vi "Module for RF and LO synthesizer.vi"(10 "Main controller mailbox":T4, 11 "THz module mailbox":T4) -> ()   [LabVIEW 2021, in "THz source modeule.lvlib"]
doc: "Module to set constant frequency or simple frequency sweep on RF (main) synthesizer and offset frequency on LO (folowing) synthesizer.\nKey typedefs: THz_Message for module, THz_Comands enum (Ignore, Initialize, Update, Set parameters, Disconnect, End), THz_Sweeep parameters\n\nComands and responses:\nInitialize: VDI config constants {Master{lower limit, upper limit, name, handle, description}, Follower{ lower limit, upper limit, name, handle, description } } (cluster of two clusters {numeric, numeric, string, numeric, string}) / handle log (string)\nUpdate: - / M_ID F_ID (string)\nSet parameters: Sweep parameters {Start, End, Sweep up time, Sweep down time, Intermediate, Reset trigger} (cluster{numeric, numeric, numeric, numeric, numeric, boolean}) / Sweep parameters (same cluster)\nDisconnect: - / master and follower name (string)\nEnd: - / Master and Follower handle (string)"
uses:
  THz source modeule.lvlib
  Messenger service/Data types/Mailbox address.ctl
  ctl/VDI config constants.ctl
  ctl/Synth configs.ctl
  ctl/THz sweep parameters.ctl
  Messenger service/Data types/Module name.ctl
  ctl/THz Message for module.ctl
  ctl/THz commands enum.ctl
  <vilib>/Utility/error.llb/Error Cluster From Error Code.vi
  <vilib>/ErrorRing/Error Ring.xnode
  Messenger service/MessengerLib.lvlib
panel:
  out "FT_Status_Update_Master":u32(ring) items=["FT_OK", "FT_INVALID_HANDLE", "FT_DEVICE_NOT_FOUND", "FT_DEVICE_NOT_OPENED", "FT_IO_ERROR", "FT_INSUFFICIENT_RESOURCES", "FT_INVALID_PARAMETER", "FT_INVALID_BAUD_RATE", "FT_DEVICE_NOT_OPENED_FOR_ERASE", "FT_DEVICE_NOT_OPENED_FOR_WRITE", "FT_FAILED_TO_WRITE_DEVICE", "FT_EEPROM_READ_FAILED", "FT_EEPROM_WRITE_FAILED", "FT_EEPROM_ERASE_FAILED", "FT_EEPROM_NOT_PRESENT", "FT_EEPROM_NOT_PROGRAMMED", "FT_INVALID_ARGS", "FT_NOT_SUPPORTED", "FT_OTHER_ERROR"]
  out "Sweep parameters":T1={"Start [GHz]"=8.0, "End [GHz] "=8.0, "Sweep up\ntime [ms]"=0.0, "Sweep down\ntime [ms]"=0.0, "Intermidiate [MHz]"=0.0, "Reset trigger"=FALSE} {"Sweep down\ntime [ms]" min=0.0 max=250.0; "End [GHz]" min=8.0 max=20.0; "Intermidiate [MHz]" min=0.0 max=2500.0; "Start [GHz]" min=8.0 max=20.0}
  out "FT_Status Update F":u32(ring) items=["FT_OK", "FT_INVALID_HANDLE", "FT_DEVICE_NOT_FOUND", "FT_DEVICE_NOT_OPENED", "FT_IO_ERROR", "FT_INSUFFICIENT_RESOURCES", "FT_INVALID_PARAMETER", "FT_INVALID_BAUD_RATE", "FT_DEVICE_NOT_OPENED_FOR_ERASE", "FT_DEVICE_NOT_OPENED_FOR_WRITE", "FT_FAILED_TO_WRITE_DEVICE", "FT_EEPROM_READ_FAILED", "FT_EEPROM_WRITE_FAILED", "FT_EEPROM_ERASE_FAILED", "FT_EEPROM_NOT_PRESENT", "FT_EEPROM_NOT_PROGRAMMED", "FT_INVALID_ARGS", "FT_NOT_SUPPORTED", "FT_OTHER_ERROR"]
  out "Ended":bool
  out "Constants":T2={"Master"={"Lower limit [GHz]"=9.0, "Upper limit [GHz]"=15.0, "Name"="VDIS0122", "Handle"=0, "Description"="VDI Synth"}, "Follower"={"Lower limit [GHz]"=9.0, "Upper limit [GHz]"=15.0, "Name"="VDIYT7", "Handle"=0, "Description"="VDI Tracking"}}
  out "Connected":bool
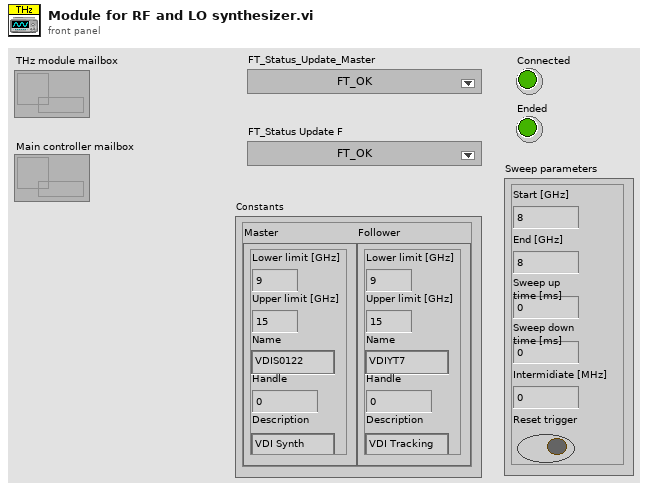
[diagram p1: front panel]
types:
  T1 = typedef "THz source modeule.lvlib/THz sweep parameters.ctl" = cluster{"Start [GHz]":dbl, "End [GHz] ":dbl, "Sweep up\ntime [ms]":dbl, "Sweep down\ntime [ms]":dbl, "Intermidiate [MHz]":dbl, "Reset trigger":bool}
  T2 = typedef "VDI config constants.ctl" = cluster{"Master":T3, "Follower":T3}
  T3 = typedef "THz source modeule.lvlib/Synth configs.ctl" = cluster{"Lower limit [GHz]":dbl, "Upper limit [GHz]":dbl, "Name":string, "Handle":u32, "Description":string}
  T4 = typedef "MessengerLib.lvlib/Mailbox address.ctl" = refnum<queue>
  T5 = typedef "THz source modeule.lvlib/THz Message for module.ctl" = cluster{"Command":T6, "Data":variant}
  T6 = typedef "THz source modeule.lvlib/THz commands enum.ctl" = enum16{"Ignore", "Initialize", "Update", "Set parameters", "Disconnect", "End"}
  T7 = typedef "Module name.ctl" = enum16{"Emty", "Magnet", "VTI", "Excitation", "Servo", "Acquisition", "Rotator", "Digitizer", "SMU2450", "Carousel", "Multimeter", "Tmp monitor", "Power monitor"}
  T8 = typedef "THz source modeule.lvlib/VDI status.ctl" = cluster{"Master":T9, "Follower":T9}
  T9 = typedef "THz source modeule.lvlib/Synth status.ctl" = cluster{"Mode":enum16{"CW", "Sweep"}, "Conected":bool}
  T10 = cluster{"Type":u32, "VID":string, "PID":string, "Serial Number":string, "Description":string}
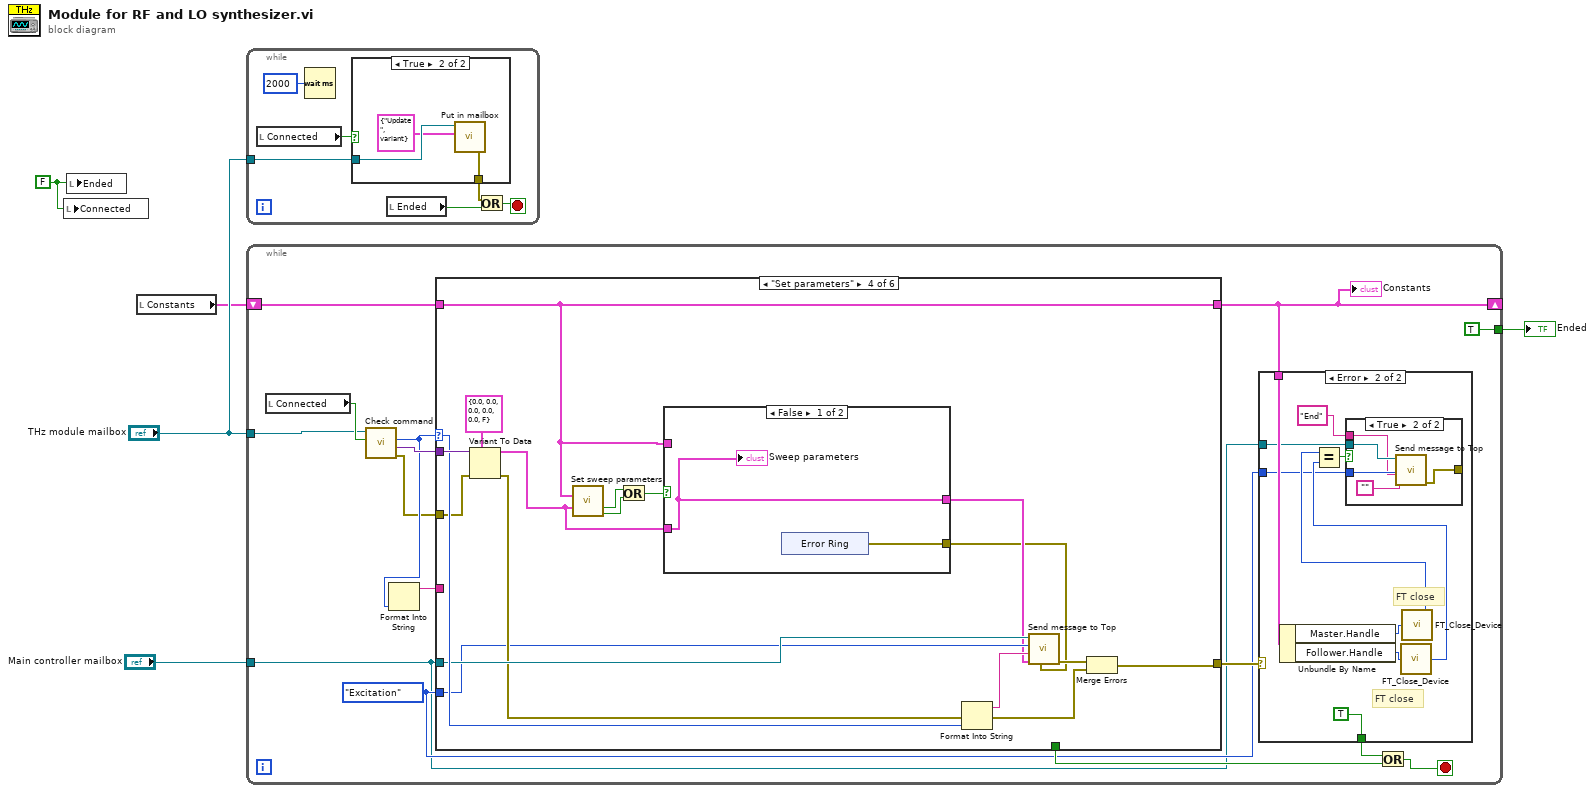
[diagram p0: block diagram]
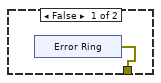
[diagram p2: hidden frame]
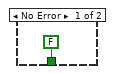
[diagram p3: hidden frame]
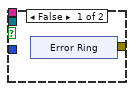
[diagram p4: hidden frame]
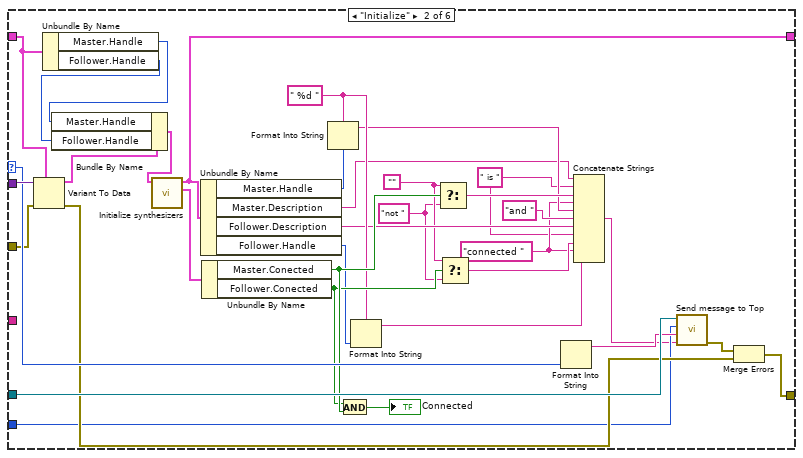
[diagram p6: hidden frame]
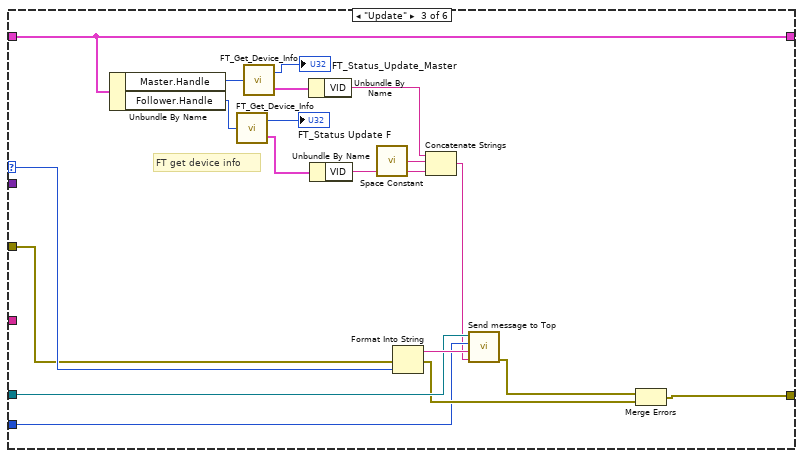
[diagram p7: hidden frame]
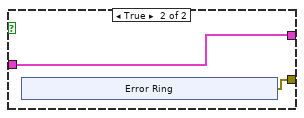
[diagram p8: hidden frame]
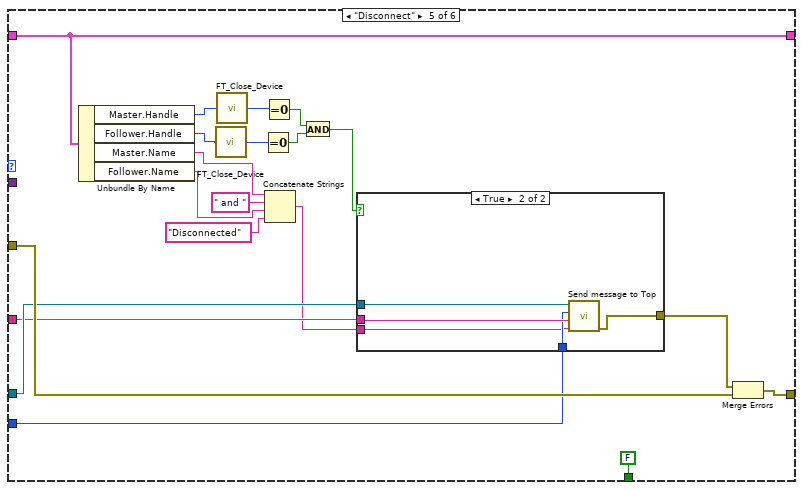
[diagram p9: hidden frame]
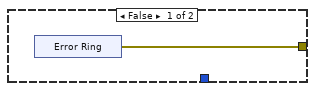
[diagram p10: hidden frame]
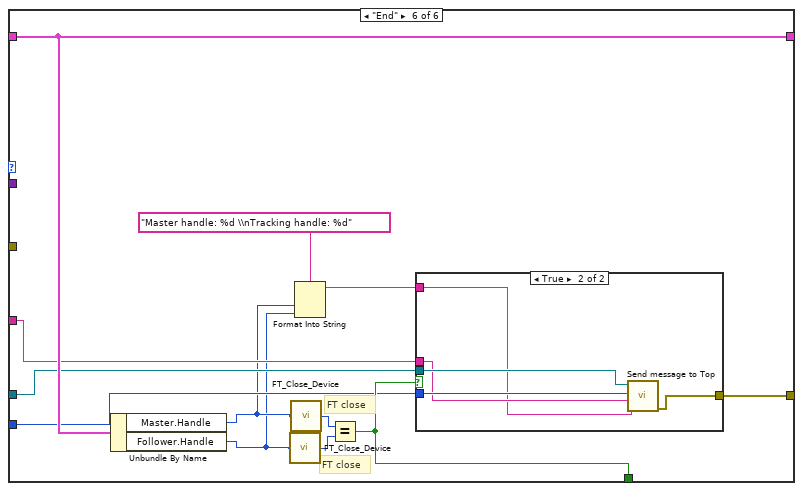
[diagram p11: hidden frame]
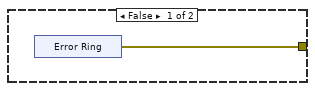
[diagram p12: hidden frame]
diagram:
  w1 = FALSE ("Initialized")
  n1 = local write "Connected"(w1) -> ()
  n2 = local write "Ended"(w1) -> ()
  n3 = local read "Constants"() -> (w3:T2)
  n4 = while {
    tunnel: "THz module mailbox" -> [w9]
    stop <- w8 stop-if-true
    n5 = local read "Connected"() -> (w10:bool)
    n6 = Wait (ms)(milliseconds to wait=u32 2000) -> ()  [unwired: 1 out]
    n7 = case shown="True" w10 {
      tunnel: w9 -> [_ w16]
      tunnel: [w12 w14] -> w7
      frame False {
        n8 = xnode "Error Ring"() -> ("error out"=w12:errorcluster)
      }
      frame True {
        n9 = call "Put in mailbox.vi"("Message"=T5 {"Command"=enum."Update", "Data"=variant} ("Incoming msg"), "Queue in"=w16) -> ("error out"=w14:errorcluster)  [unwired: 7 in, 2 out]
      }
    }
    n10 = local read "Ended"() -> (w6:bool)
    n11 = Or(x=w7, y=w6) -> (x .or. y?=w8:bool)
  }
  n12 = while {
    shift-right: [w28] -> _
    shift-left: w3 -> [w31]
    tunnel: "THz module mailbox" -> [w20]
    tunnel: "Main controller mailbox" -> [w17]
    tunnel: [TRUE ("Initialized")] -> w2
    stop <- w26 stop-if-true
    w18 = Module_name."Excitation" ("Module")
    n13 = local read "Connected"() -> (w29:bool)
    n14 = call "Check command.vi"("Is initialized"=w29, "Module mailbox"=w20) -> ("error out"=w19:errorcluster, "Command Data"=w30:variant, "Command"=w22:T6)  [unwired: 3 in]
    n15 = Format Into String(w22) -> (resulting string=w21:string)  [unwired: 3 in, 1 out]
    n16 = case shown="\"Set parameters\"" w22 {
      selector: w22 -> [_ w83 w103 w119 _ _]
      tunnel: [w51 w72 w97 w106 w147 w170] -> w28
      tunnel: w31 -> [w51 w54 w97 w106 w147 w170]
      tunnel: w30 -> [_ w85 _ w122 _ _]
      tunnel: [_ _ _ _ FALSE w168] -> w27
      tunnel: w17 -> [_ w82 w102 w117 w146 w169]
      tunnel: [w50 w78 w100 w113 w150 w167] -> w23
      tunnel: w19 -> [w50 w76 w99 w115 w151 _]
      tunnel: w18 -> [_ w70 w96 w110 w139 w163]
      tunnel: w21 -> [_ _ _ _ w140 w166]
      frame "Ignore", Default {
      }
      frame "Initialize" {
        w68 = " %d " ("format string")
        w61 = ""
        w58 = " is "
        w59 = "connected "
        w60 = "not "
        n17 = Variant To Data(error in=w76, type=w54, Variant=w85) -> (data=w74:T2, error out=w75:errorcluster)
        n18 = Unbundle By Name(w54) -> ("Master.Handle"=w52:u32, "Follower.Handle"=w53:u32)
        n19 = Bundle By Name(cluster=w74, "Master.Handle"=w52, "Follower.Handle"=w53) -> (w55:T2)
        n20 = call "Initialize synthesizers.vi"("VDI config constants in"=w55) -> ("Status"=w73:T8, "VDI config constants out"=w72:T2)  [unwired: 9 in]
        n21 = Unbundle By Name(w72) -> ("Master.Handle"=w57:u32, "Master.Description"=w66:string, "Follower.Description"=w64:string, "Follower.Handle"=w56:u32)
        n22 = Unbundle By Name(w73) -> ("Master.Conected"=w79:bool, "Follower.Conected"=w71:bool)
        n23 = Format Into String(format string=w68, w57) -> (resulting string=w67:string)  [unwired: 2 in, 1 out]
        n24 = And(x=w71, y=w79) -> (x .and. y?=→"Connected":bool)
        n25 = Format Into String(format string=w68, w56) -> (resulting string=w62:string)  [unwired: 2 in, 1 out]
        n26 = Select(t=w61, s=w79, f=w60) -> (s? t:f=w84:string)
        n27 = Select(t=w61, s=w71, f=w60) -> (s? t:f=w63:string)
        n28 = Format Into String(w83) -> (resulting string=w81:string)  [unwired: 3 in, 1 out]
        n29 = Concatenate Strings(w66, w58, w84, w59, w67, "and ", w64, w58, w63, w59, w62) -> (w69:string)
        n30 = call "Send message to Top.vi"("Data"=w69, "Response"=w81, "Module"=w70, "Mailbox address in"=w82) -> ("Error out"=w77:errorcluster)  [unwired: 6 in, 1 out]
        n31 = Merge Errors(w77, w75) -> (w78:errorcluster)
      }
      frame "Update" {
        # "FT get device info"
        n32 = Unbundle By Name(w97) -> ("Master.Handle"=w92:u32, "Follower.Handle"=w95:u32)
        n33 = call <instrlib>:"FT_Get_Device_Info.vi"("Handle"=w95) -> ("FT_Status"=→"FT_Status Update F":u32, "Device Information"=w94:T10)
        n34 = call <instrlib>:"FT_Get_Device_Info.vi"("Handle"=w92) -> ("FT_Status"=→"FT_Status_Update_Master":u32, "Device Information"=w91:T10)
        n35 = Unbundle By Name(w91) -> ("VID"=w89:string)
        n36 = Unbundle By Name(w94) -> ("VID"=w93:string)
        n37 = call <vilib>:"Space Constant.vi"() -> ("String"=w88:string)
        n38 = Format Into String(error in=w99, w103) -> (resulting string=w104:string, error out=w98:errorcluster)  [unwired: 2 in]
        n39 = Concatenate Strings(w89, w88, w93) -> (w90:string)
        n40 = call "Send message to Top.vi"("Data"=w90, "Response"=w104, "Module"=w96, "Mailbox address in"=w102) -> ("Error out"=w101:errorcluster)  [unwired: 6 in, 1 out]
        n41 = Merge Errors(w101, w98) -> (w100:errorcluster)
      }
      frame "Set parameters" {
        n42 = Variant To Data(error in=w115, type=T1 {"Start [GHz]"=0.0, "End [GHz] "=0.0, "Sweep up\ntime [ms]"=0.0, "Sweep down\ntime [ms]"=0.0, "Intermidiate [MHz]"=0.0, "Reset trigger"=FALSE} ("Sweep parameters"), Variant=w122) -> (data=w107:T1, error out=w114:errorcluster)
        n43 = call "Set sweep parameters.vi"("VDI config constants"=w106, "Sweep parameters"=w107) -> ("Error1"=w118:bool, "Error2"=w116:bool)  [unwired: 9 in, 3 out]
        n44 = Or(x=w118, y=w116) -> (x .or. y?=w109:bool)
        n45 = case shown="False" w109 {
          tunnel: [w124 w126] -> w108
          tunnel: w107 -> [w124 w126]
          tunnel: w106 -> [_ _]
          tunnel: [w123 w127] -> w105
          frame False {
            n46 = xnode "Error Ring"() -> ("error out"=w123:errorcluster)
            "Sweep parameters" <- w124
          }
          frame True {
            n47 = xnode "Error Ring"() -> ("error out"=w127:errorcluster)
          }
        }
        n48 = Format Into String(error in=w114, w119) -> (resulting string=w120:string, error out=w112:errorcluster)  [unwired: 2 in]
        n49 = call "Send message to Top.vi"("Error in (no error)"=w105, "Data"=w108, "Response"=w120, "Module"=w110, "Mailbox address in"=w117) -> ("Error out"=w111:errorcluster)  [unwired: 5 in, 1 out]
        n50 = Merge Errors(w111, w112) -> (w113:errorcluster)
      }
      frame "Disconnect" {
        n51 = Unbundle By Name(w147) -> ("Master.Handle"=w149:u32, "Follower.Handle"=w148:u32, "Master.Name"=w138:string, "Follower.Name"=w137:string)
        n52 = call <instrlib>:"FT_Close_Device.vi"("Handle"=w148) -> ("FT_Status"=w144:u32)
        n53 = call <instrlib>:"FT_Close_Device.vi"("Handle"=w149) -> ("FT_Status"=w143:u32)
        n54 = Equal To 0?(x=w144) -> (x = 0?=w145:bool)
        n55 = Equal To 0?(x=w143) -> (x = 0?=w142:bool)
        n56 = Concatenate Strings(w138, " and " ("string"), w137, "Disconnected" ("string")) -> (w132:string)
        n57 = And(x=w142, y=w145) -> (x .and. y?=w141:bool)
        n58 = case shown="True" w141 {
          tunnel: w146 -> [_ w158]
          tunnel: [w152 w157] -> w134
          tunnel: w140 -> [_ w156]
          tunnel: w139 -> [_ w155]
          tunnel: w132 -> [_ w154]
          frame False {
            n59 = xnode "Error Ring"() -> ("error out"=w152:errorcluster)
          }
          frame True {
            n60 = call "Send message to Top.vi"("Data"=w154, "Response"=w156, "Module"=w155, "Mailbox address in"=w158) -> ("Error out"=w157:errorcluster)  [unwired: 6 in, 1 out]
          }
        }
        n61 = Merge Errors(w134, w151) -> (w150:errorcluster)
      }
      frame "End" {
        # "FT close"
        # "FT close"
        n62 = Unbundle By Name(w170) -> ("Master.Handle"=w161:u32, "Follower.Handle"=w160:u32)
        n63 = call <instrlib>:"FT_Close_Device.vi"("Handle"=w160) -> ("FT_Status"=w164:u32)
        n64 = call <instrlib>:"FT_Close_Device.vi"("Handle"=w161) -> ("FT_Status"=w165:u32)
        n65 = Format Into String(format string="Master handle: %d \\nTracking handle: %d", w161, w160) -> (resulting string=w159:string)  [unwired: 2 in, 1 out]
        n66 = Equal?(x=w165, y=w164) -> (x = y?=w168:bool)
        n67 = case shown="True" w168 {
          tunnel: w169 -> [_ w177]
          tunnel: [w171 w176] -> w167
          tunnel: w163 -> [_ w175]
          tunnel: w166 -> [_ w174]
          tunnel: w159 -> [_ w173]
          frame False {
            n68 = xnode "Error Ring"() -> ("error out"=w171:errorcluster)
          }
          frame True {
            n69 = call "Send message to Top.vi"("Data"=w173, "Response"=w174, "Module"=w175, "Mailbox address in"=w177) -> ("Error out"=w176:errorcluster)  [unwired: 6 in, 1 out]
          }
        }
      }
    }
    "Constants" <- w28
    n70 = case shown="Error" w23 {
      tunnel: w28 -> [_ w42]
      tunnel: [FALSE TRUE] -> w25
      tunnel: w18 -> [_ w34]
      tunnel: w17 -> [_ w33]
      frame No Error {
      }
      frame Error {
        # "FT close"
        # "FT close"
        n71 = Unbundle By Name(w42) -> ("Master.Handle"=w40:u32, "Follower.Handle"=w39:u32)
        n72 = call <instrlib>:"FT_Close_Device.vi"("Handle"=w39) -> ("FT_Status"=w35:u32)
        n73 = call <instrlib>:"FT_Close_Device.vi"("Handle"=w40) -> ("FT_Status"=w36:u32)
        n74 = Equal?(x=w36, y=w35) -> (x = y?=w38:bool)
        n75 = case shown="True" w38 {
          tunnel: w33 -> [_ w49]
          tunnel: [w43 w48] -> _
          tunnel: w34 -> [_ w46]
          tunnel: "End" -> [_ w45]
          frame False {
            n76 = xnode "Error Ring"() -> ("error out"=w43:errorcluster)
          }
          frame True {
            n77 = call "Send message to Top.vi"("Data"="", "Response"=w45, "Module"=w46, "Mailbox address in"=w49) -> ("Error out"=w48:errorcluster)  [unwired: 6 in, 1 out]
          }
        }
      }
    }
    n78 = Or(x=w25, y=w27) -> (x .or. y?=w26:bool)
  }
  "Ended" <- w2
